vi "SetAxisSpaceCfg.vi"(5 "Axis Space Config":T1, 11 "error in (no error)":errorcluster) -> (15 "error out":errorcluster)   [LabVIEW 2009]
doc: "Sets limit parameters for each axis."
uses:
  typedefs/AxisSpaceCfg.ctl
  typedefs/AxisCfg.ctl
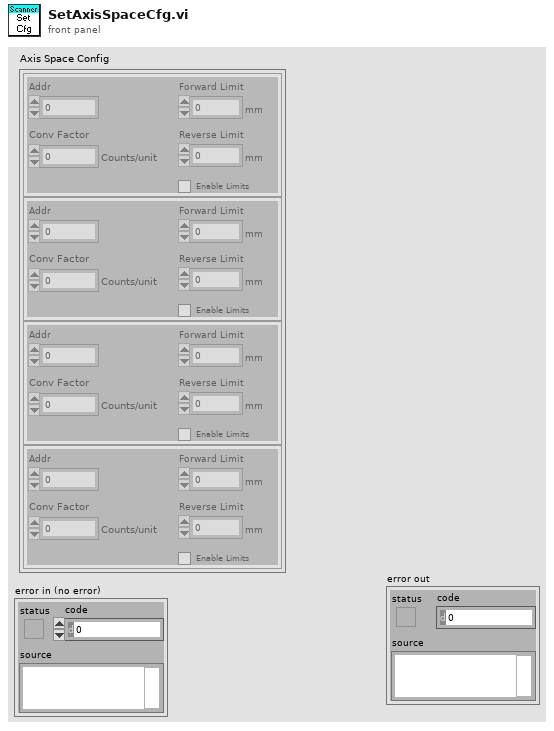
[diagram p1: front panel]
types:
  T1 = typedef "AxisSpaceCfg.ctl" = T2[]
  T2 = typedef "AxisCfg.ctl" = cluster{"Addr":u8, "Conv Factor":dbl, "Forward Limit":dbl, "Reverse Limit":dbl, "Enable Limits":bool}
  T3 = typedef "AxisSelect_Enum.ctl" = enum16{"X", "Y", "Z", "Axis Space"}
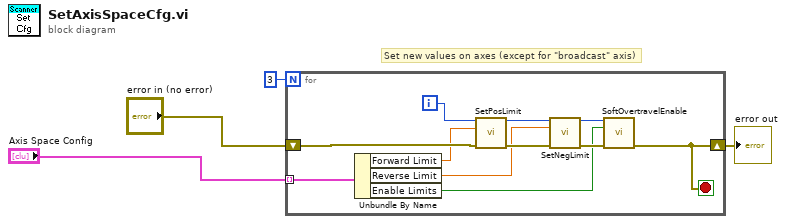
[diagram p0: block diagram]
diagram:
  # "Set new values on axes (except for \"broadcast\" axis)"
  n1 = for {
    N: 3 -> [_]
    tunnel: "Axis Space Config" -> [w15] mode=indexing
    shift-right: [w8] -> w2
    shift-left: "error in (no error)" -> [w12]
    i -> [w14]
    stop <- w8 stop-if-true
    n2 = Unbundle By Name(w15) -> ("Forward Limit"=w7:dbl, "Reverse Limit"=w6:dbl, "Enable Limits"=w5:bool)
    n3 = call "SetPosLimit.vi"("Axis In"=w14, "Positive Limit"=w7, "error in (no error)"=w12) -> ("Axis Out"=w13:T3, "error out"=w11:errorcluster)  [unwired: 11 in]
    n4 = call "SetNegLimit.vi"("Axis In"=w13, "Negative Limit"=w6, "error in (no error)"=w11) -> ("Axis Out"=w9:T3, "error out"=w10:errorcluster)  [unwired: 11 in]
    n5 = call "SoftOvertravelEnable.vi"("Axis In"=w9, "Enable (T)"=w5, "error in (no error)"=w10) -> ("error out"=w8:errorcluster)  [unwired: 11 in, 1 out]
  }
  "error out" <- w2
